vi "T Test.vi"(6 "alternative hypothesis":i32(ring) items=["mean(pop) != mean"=0, "mean(pop) > mean"=1, "mean(pop) < mean"=-1], 9 "significance level":dbl=0.05, 10 "mean":dbl, 11 "sample set":dbl[](array[numeric])) -> (0 "error":i32, 1 "confidence interval":cluster{"low":dbl, "high":dbl}={"low"=0.8260722090132093, "high"=0.8260722090132093} {"high" format="%.6g"; "low" format="%.6g"}, 2 "p value":dbl=0.05 format="%.6g", 3 "reject null hypothesis":bool, 4 "t test info":T1 {"sample t value" format="%_6g"; "t value" format="%_6g"; "sample se mean" format="%_6g"; "sample std" format="%_6g"; "sample mean" format="%_6g"})   [LabVIEW 2014, in "NI_Gmath.lvlib"]
doc: "Tests hypotheses about the <B>mean</B> of a population whose distribution is at least approximately normal but whose variance is unknown."
uses:
  NI_Gmath.lvlib
  st_t_control.ctl
  NI_AALBase.lvlib
panel:
  # "T Test\n(single sample set)"
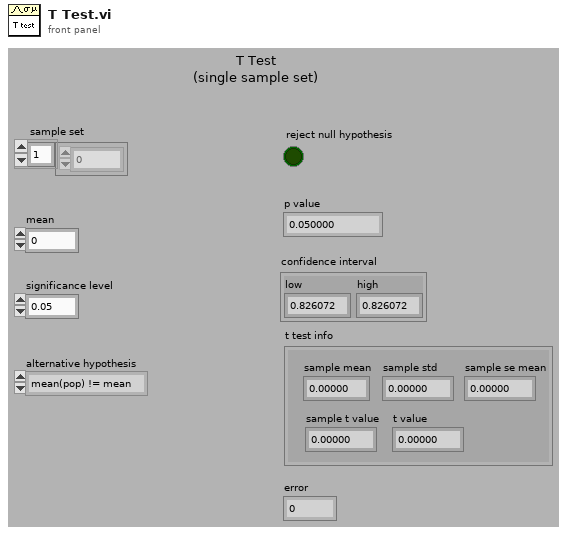
[diagram p1: front panel]
types:
  T1 = typedef "NI_Gmath.lvlib/st_t_control.ctl" = cluster{"sample mean":dbl, "sample std":dbl, "sample se mean":dbl, "sample t value":dbl, "t value":dbl}
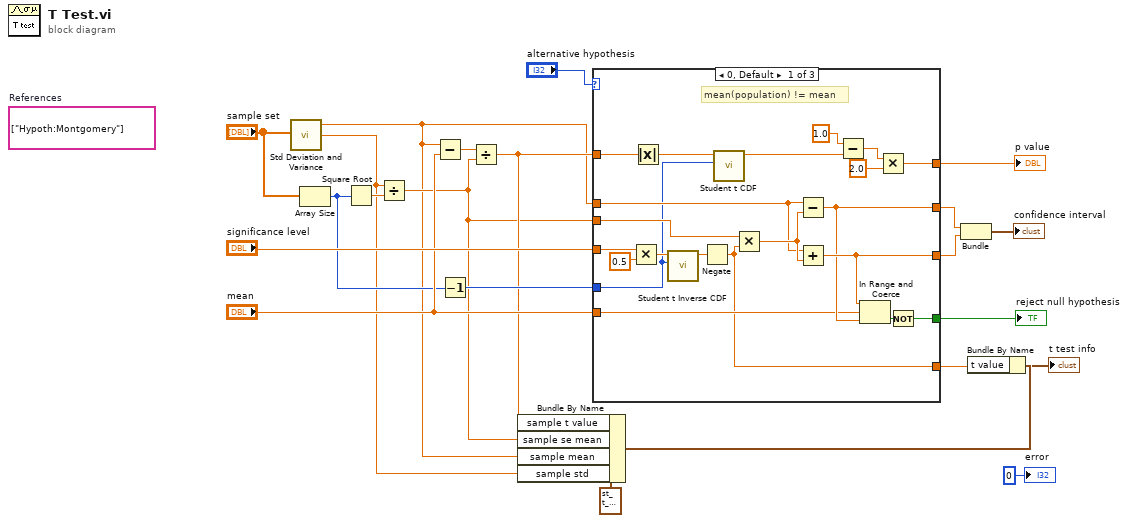
[diagram p0: block diagram]
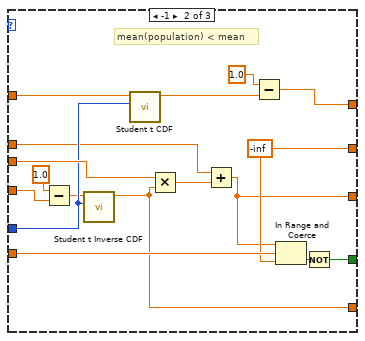
[diagram p2: hidden frame]
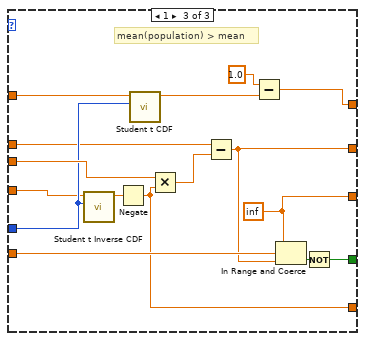
[diagram p3: hidden frame]
diagram:
  (unwired) string[] ["Hypoth:Montgomery"]  # References
  n1 = call "Std Deviation and Variance.vi"("X"="sample set") -> ("mean"=w1:dbl, "standard deviation"=w9:dbl)  [unwired: 1 in, 1 out]
  n2 = Array Size(array="sample set") -> (size(s)=w10:i32)
  n3 = Square Root(x=w10) -> (sqrt(x)=w11:dbl)
  n4 = Divide(x=w9, y=w11) -> (x/y=w7:dbl)
  n5 = Subtract(x=w1, y="mean") -> (x-y=w21:dbl)
  n6 = Decrement(x=w10) -> (x-1=w18:i32)
  n7 = Divide(x=w21, y=w7) -> (x/y=w8:dbl)
  n8 = Bundle By Name(cluster=T1 {"sample mean"=0.0, "sample std"=0.0, "sample se mean"=0.0, "sample t value"=0.0, "t value"=0.0} ("t test info"), "sample t value"=w8, "sample se mean"=w7, "sample mean"=w1, "sample std"=w9) -> (w6:T1)
  n9 = case shown="0, Default" "alternative hypothesis" {
    tunnel: "significance level" -> [w42 w49 w67]
    tunnel: w18 -> [w31 w56 w71]
    tunnel: w7 -> [w41 w60 w76]
    tunnel: [w37 w44 w64] -> w17
    tunnel: [w36 w45 w65] -> w16
    tunnel: [w34 w57 w73] -> w15
    tunnel: "mean" -> [w33 w52 w72]
    tunnel: w1 -> [w32 w51 w66]
    tunnel: w8 -> [w30 w46 w70]
    tunnel: [w25 w53 w63] -> w12
    tunnel: [w24 w47 w61] -> w4
    frame 0, Default {
      # "mean(population) != mean"
      n10 = Multiply(x=w42, y=0.5) -> (x*y=w38:dbl)
      n11 = Absolute Value(x=w30) -> (abs(x)=w23:dbl)
      n12 = call "Student t Inverse CDF.vi"("k degrees of freedom"=w31, "cdf(x)"=w38) -> ("x"=w39:dbl)  [unwired: 8 in, 1 out]
      n13 = Negate(x=w39) -> (-x=w24:dbl)
      n14 = call "Student t CDF.vi"("k degrees of freedom"=w31, "x"=w23) -> ("cdf(x)"=w28:dbl)  [unwired: 7 in, 2 out]
      n15 = Multiply(x=w41, y=w24) -> (x*y=w40:dbl)
      n16 = Subtract(x=w32, y=w40) -> (x-y=w36:dbl)
      n17 = Add(x=w32, y=w40) -> (x+y=w37:dbl)
      n18 = Subtract(x=1.0, y=w28) -> (x-y=w26:dbl)
      n19 = In Range and Coerce(upper limit=w37, x=w33, lower limit=w36) -> (In Range?=w35:bool)  [unwired: 1 out]
      n20 = Multiply(x=w26, y=2.0) -> (x*y=w25:dbl)
      n21 = Not(x=w35) -> (.not. x?=w34:bool)
    }
    frame -1 {
      w45 = -inf ("lower limit")
      # "mean(population) < mean"
      n22 = Subtract(x=1.0, y=w49) -> (x-y=w48:dbl)
      n23 = call "Student t Inverse CDF.vi"("k degrees of freedom"=w56, "cdf(x)"=w48) -> ("x"=w47:dbl)  [unwired: 8 in, 1 out]
      n24 = call "Student t CDF.vi"("k degrees of freedom"=w56, "x"=w46) -> ("cdf(x)"=w54:dbl)  [unwired: 7 in, 2 out]
      n25 = Multiply(x=w60, y=w47) -> (x*y=w59:dbl)
      n26 = Add(x=w51, y=w59) -> (x+y=w44:dbl)
      n27 = Subtract(x=1.0, y=w54) -> (x-y=w53:dbl)
      n28 = In Range and Coerce(upper limit=w44, x=w52, lower limit=w45) -> (In Range?=w58:bool)  [unwired: 1 out]
      n29 = Not(x=w58) -> (.not. x?=w57:bool)
    }
    frame 1 {
      w64 = inf
      # "mean(population) > mean"
      n30 = call "Student t Inverse CDF.vi"("k degrees of freedom"=w71, "cdf(x)"=w67) -> ("x"=w62:dbl)  [unwired: 8 in, 1 out]
      n31 = Negate(x=w62) -> (-x=w61:dbl)
      n32 = call "Student t CDF.vi"("k degrees of freedom"=w71, "x"=w70) -> ("cdf(x)"=w68:dbl)  [unwired: 7 in, 2 out]
      n33 = Multiply(x=w76, y=w61) -> (x*y=w75:dbl)
      n34 = Subtract(x=w66, y=w75) -> (x-y=w65:dbl)
      n35 = Subtract(x=1.0, y=w68) -> (x-y=w63:dbl)
      n36 = In Range and Coerce(upper limit=w64, x=w72, lower limit=w65) -> (In Range?=w74:bool)  [unwired: 1 out]
      n37 = Not(x=w74) -> (.not. x?=w73:bool)
    }
  }
  "reject null hypothesis" <- w15
  "p value" <- w12
  n38 = Bundle("lower limit"=w16, w17) -> (→"confidence interval":cluster{"lower limit":dbl, dbl})  [unwired: 1 in]
  n39 = Bundle By Name(cluster=w6, "t value"=w4) -> (→"t test info":T1)
  "error" <- 0 ("error")
